vi "Test.vi"(0 "current":dbl, 11 "error in (no error)":errorcluster) -> (4 "voltage":dbl=24.0, 6 "measurement data":T1={"name"="Voltage Test", "measurement"=24.0, "low limit"=5.0, "high limit"=36.0, "comparison type"="GTLT", "status"="Passed", "units"="volts"}, 10 "test time":dbl, 15 "error out":errorcluster)   [LabVIEW 2018]
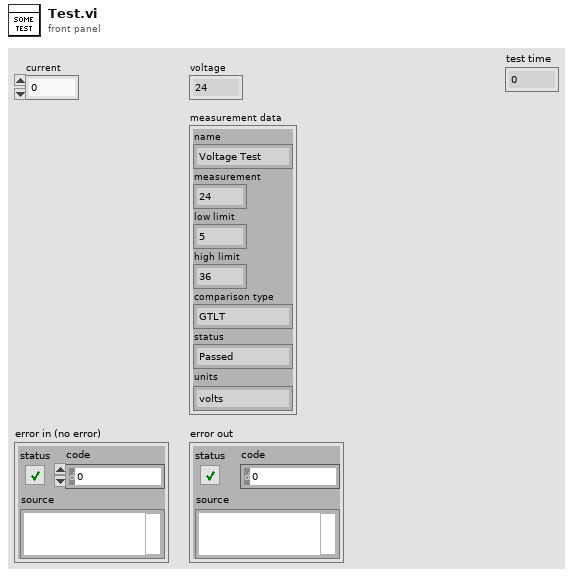
[diagram p1: front panel]
types:
  T1 = cluster{"name":string, "measurement":dbl, "low limit":dbl, "high limit":dbl, "comparison type":string, "status":string, "units":string}
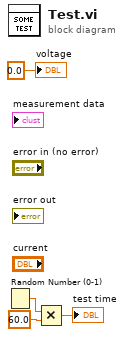
[diagram p0: block diagram]
diagram:
  n1 = Random Number (0-1)() -> (number: 0 to 1=w3:dbl)
  n2 = Multiply(x=w3, y=60.0 ("number (0 to 1)")) -> (x*y=→"test time":dbl)
  "voltage" <- 0.0 ("output")
